vi "G#Debugger_GetClassMethods.vi"(0 "LVClassLibrary Refnum":refnum<vi>, 5 "error in (no error)":errorcluster) -> (15 "method names":string[](array[string]), 17 "method paths":path[](array[path]), 19 "error out":errorcluster)   [LabVIEW 2017, in "G#Debugger.lvlib"]
uses:
  G#Debugger.lvlib
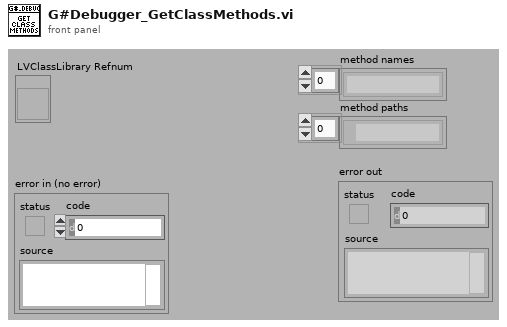
[diagram p1: front panel]
types:
  T1 = enum32{"invalid scope", "public", "private", "protected", "community"}
  T2 = enum32{"invalid VI type", "Standard VI", "Control VI", "Global VI", "Polymorphic VI", "Configuration VI", "SubSystem", "Facade VI", "Method VI", "Statechart Diagram VI"}
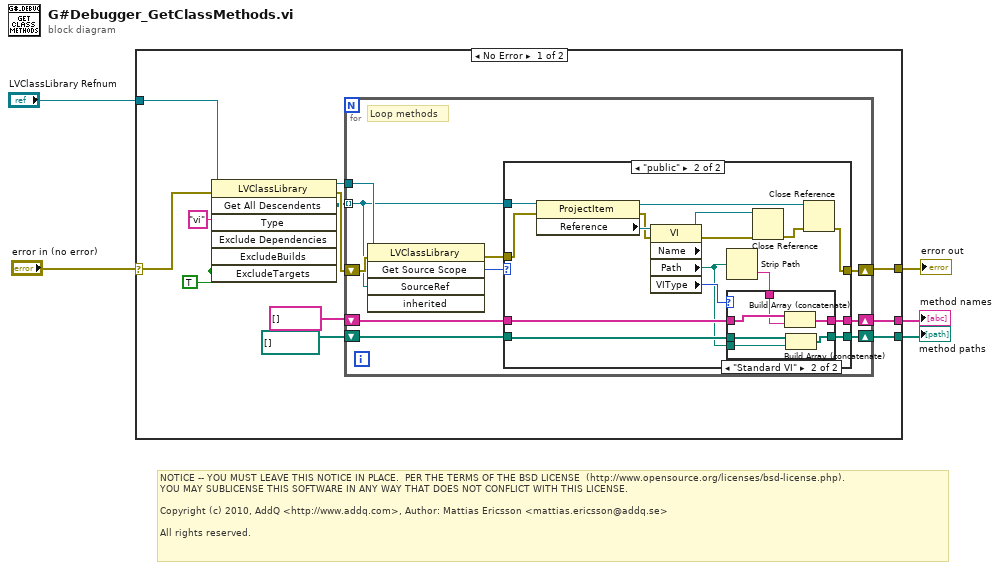
[diagram p0: block diagram]
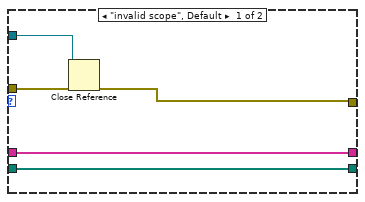
[diagram p2: hidden frame]
diagram:
  # "NOTICE -- YOU MUST LEAVE THIS NOTICE IN PLACE.  PER THE TERMS OF THE BSD LICENSE  (http://www.opensource.org/licenses/bsd-license.php).\nYOU MAY SUBLICENSE THIS SOFTWARE IN ANY WAY THAT DOES NOT CONFLICT WITH THIS LICENSE.\n\nCopyright (c) 2010, AddQ <http://www.addq.com>, Author: Mattias Ericsson <mattias.ericsson@addq.se>\n\nAll rights reserved."
  n1 = case shown="No Error" "error in (no error)" {
    selector: "error in (no error)" -> [w6 w57]
    tunnel: [w17 _] -> w5
    tunnel: [w16 _] -> w4
    tunnel: [w12 w57] -> w1
    tunnel: "LVClassLibrary Refnum" -> [w7 _]
    frame No Error {
      w9 = TRUE ("ExcludeDependencies")
      n2 = invoke class="LVClassLibrary" method="Get All Descendents"(reference=w7, error in=w6, "Type"="vi", "Exclude Dependencies"=w9, "ExcludeBuilds"=w9) -> (reference out=w13:refnum<vi>, error out=w11:errorcluster, "All Descendents"=w10:refnum<vi>[])  [unwired: 2 in, 4 out]
      n3 = for {
        tunnel: w10 -> [w23] mode=indexing
        shift-right: [w27] -> w12
        shift-left: w11 -> [w26]
        tunnel: w13 -> [w25]
        shift-right: [w20] -> w16
        shift-left: string[] [] -> [w21]
        shift-right: [w18] -> w17
        shift-left: path[] [] -> [w19]
        # "Loop methods"
        n4 = invoke class="LVClassLibrary" method="Get Source Scope"(reference=w25, error in=w26, "SourceRef"=w23) -> (error out=w24:errorcluster, "GetSourceScope"=w22:T1)  [unwired: 2 in, 3 out]
        n5 = case shown="\"public\"" w22 {
          tunnel: [w29 w42] -> w27
          tunnel: w24 -> [w30 w41]
          tunnel: w23 -> [w28 w40]
          tunnel: w21 -> [w32 w38]
          tunnel: [w32 w39] -> w20
          tunnel: w19 -> [w31 w37]
          tunnel: [w31 w36] -> w18
          frame "invalid scope", Default {
            n6 = Close Reference(reference=w28, error in (no error)=w30) -> (error out=w29:errorcluster)
          }
          frame "public" {
            n7 = property class="ProjectItem"(reference=w40, error in=w41) -> (reference out=w43:refnum<vi>, error out=w47:errorcluster, "Reference"=w48:refnum<vi>)
            n8 = property class="VI" props=["Name", "Path", "VIType"](reference=w48, error in=w47) -> (reference out=w45:refnum<vi>, error out=w46:errorcluster, "Path"=w34:path, "VIType"=w35:T2)  [unwired: 1 out]
            n9 = Strip Path(path=w34) -> (name=w33:string)  [unwired: 1 out]
            n10 = case shown="\"Standard VI\"" w35 {
              tunnel: [w50 w56] -> w39
              tunnel: w38 -> [w50 w55]
              tunnel: w33 -> [_ w54]
              tunnel: w34 -> [_ w53]
              tunnel: w37 -> [w49 w52]
              tunnel: [w49 w51] -> w36
              frame "invalid VI type", Default {
              }
              frame "Standard VI" {
                n11 = Build Array (concatenate)(w55, w54) -> (w56:string[])
                n12 = Build Array (concatenate)(w52, w53) -> (w51:path[])
              }
            }
            n13 = Close Reference(reference=w45, error in (no error)=w46) -> (error out=w44:errorcluster)
            n14 = Close Reference(reference=w43, error in (no error)=w44) -> (error out=w42:errorcluster)
          }
        }
      }
    }
    frame Error {
    }
  }
  "method paths" <- w5
  "method names" <- w4
  "error out" <- w1
